vi "FL Gaussian COA Single Side.vi"(0 "weight":dbl, 5 "Implication":T1 items=["Minimum", "Product"]) -> (4 "xlh":dbl, 6 "area":dbl, 8 "coa_x":dbl, 10 "x_l":dbl=-2.5, 15 "x_r":dbl)   [LabVIEW 2017, in "NI_Fuzzy_Logic_API.lvlib"]
uses:
  <vilib>/addons/Fuzzy Logic/NI_Fuzzy_Logic_API.lvlib
  <vilib>/addons/Fuzzy Logic/TypeDefs/FL Consequent Implication.ctl
  <vilib>/gmath/NI_Gmath.lvlib
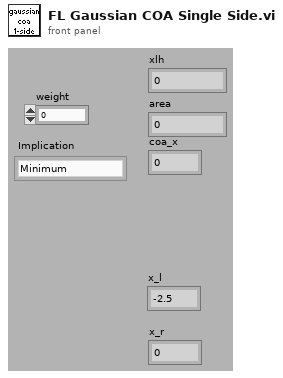
[diagram p1: front panel]
types:
  T1 = typedef "NI_Fuzzy_Logic_API.lvlib/FL Consequent Implication.ctl" = u16
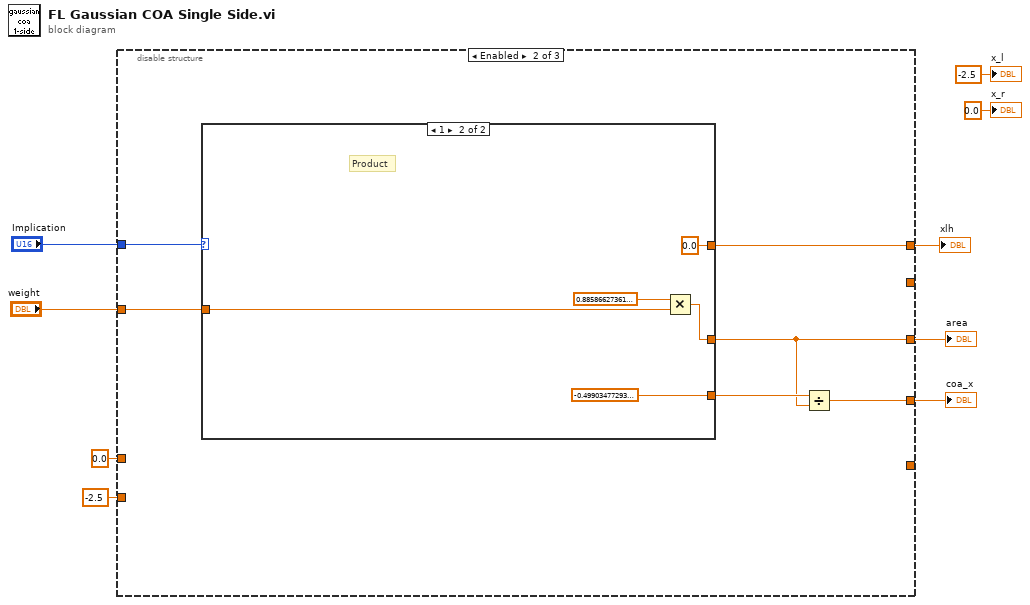
[diagram p0: block diagram]
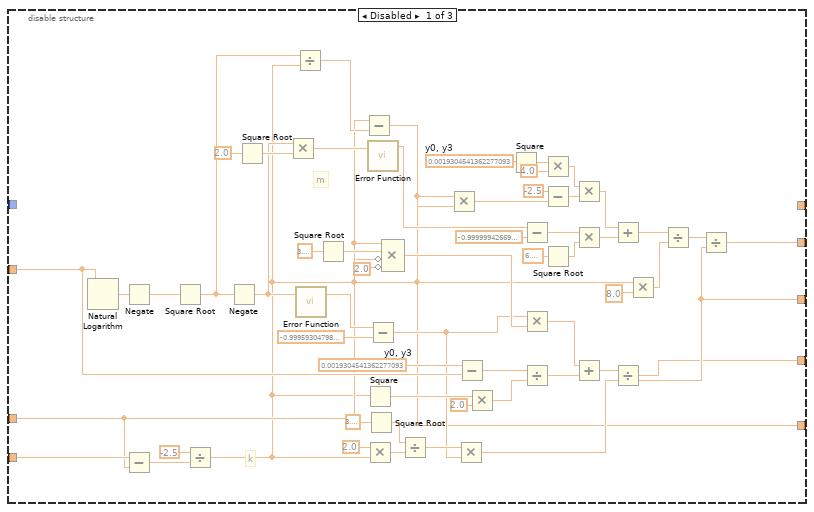
[diagram p2: hidden frame]
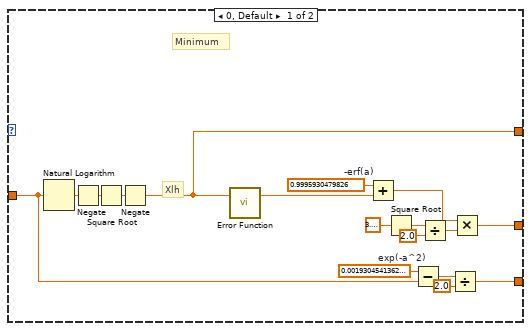
[diagram p3: hidden frame]
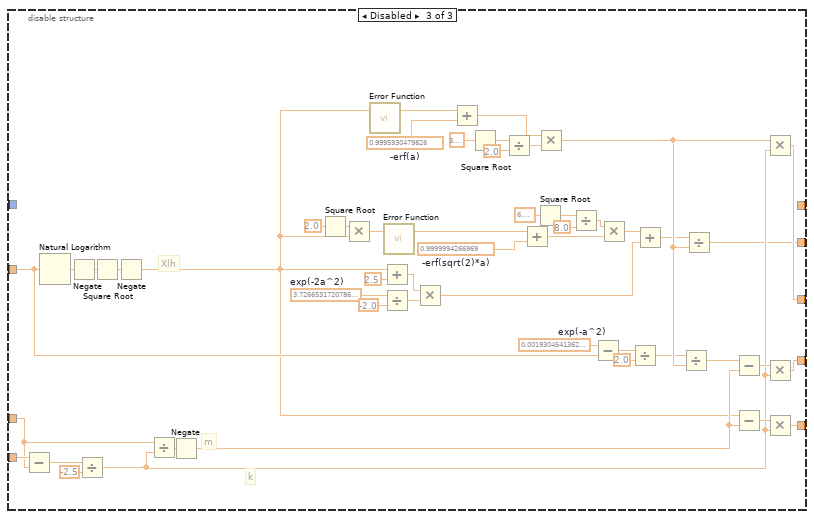
[diagram p4: hidden frame]
diagram:
  n1 = disable-structure shown="Enabled" {
    disable-tunnel: "weight" -> [w65 w70 w111]
    disable-tunnel: [w61 w69 w99] -> w8
    disable-tunnel: [w59 _ w96] -> _
    disable-tunnel: -2.5 ("x0") -> [w27 _ w133]
    disable-tunnel: 0.0 ("x1") -> [w15 _ w124]
    disable-tunnel: [w14 w68 w114] -> w7
    disable-tunnel: [w10 _ w121] -> _
    disable-tunnel: "Implication" -> [_ w67 _]
    disable-tunnel: [_ w66 _] -> w1
    frame Disabled {
      w13 = 0.0019304541362277093  # y0, y3
      w47 = 0.0019304541362277093  # y0, y3
      # "m"
      # "k"
      n2 = Natural Logarithm(1:w65) -> (0:w19:dbl)
      n3 = Negate(x=w19) -> (-x=w20:dbl)
      n4 = Subtract(x=w27, y=w15) -> (x-y=w18:dbl)
      n5 = Square Root(x=w20) -> (sqrt(x)=w64:dbl)
      n6 = Divide(x=-2.5, y=w18) -> (x/y=w12:dbl)
      n7 = Negate(x=w64) -> (-x=w38:dbl)
      n8 = Square Root(x=2.0) -> (sqrt(x)=w41:dbl)
      n9 = Multiply(x=w38, y=w41) -> (x*y=w40:dbl)
      n10 = Divide(x=w64, y=w12) -> (x/y=w21:dbl)
      n11 = call <vilib>:"Error Function.vi"("x"=w38) -> ("erf(x)"=w22:dbl)  [unwired: 2 out]
      n12 = Square Root(x=3.141592653589793) -> (sqrt(x)=w29:dbl)
      n13 = Subtract(x=w15, y=w21) -> (x-y=w10:dbl)
      n14 = Square(x=w12) -> (x^2=w32:dbl)
      n15 = Multiply(x=2.0, y=w12) -> (x*y=w25:dbl)
      n16 = Square Root(x=3.141592653589793) -> (sqrt(x)=w62:dbl)
      n17 = call <vilib>:"Error Function.vi"("x"=w40) -> ("erf(x)"=w42:dbl)  [unwired: 2 out]
      n18 = Subtract(x=w22, y=-0.999593047982555 ("erf(x)")) -> (x-y=w11:dbl)
      n19 = Compound Arithmetic op=MULTIPLY(w15, w29, invert w12, invert 2.0 ("value")) -> (w31:dbl)
      n20 = Divide(x=w62, y=w25) -> (x/y=w26:dbl)
      n21 = Multiply(x=w10, y=w12) -> (x*y=w51:dbl)
      n22 = Multiply(x=w26, y=w11) -> (x*y=w61:dbl)
      n23 = Subtract(x=w13, y=w65) -> (x-y=w34:dbl)
      n24 = Multiply(x=w32, y=2.0) -> (x*y=w35:dbl)
      n25 = Square(x=w47) -> (x^2=w48:dbl)
      n26 = Subtract(x=w42, y=-0.9999994266968563 ("erf(x)")) -> (x-y=w45:dbl)
      n27 = Multiply(x=w11, y=w31) -> (x*y=w37:dbl)
      n28 = Divide(x=w34, y=w35) -> (x/y=w36:dbl)
      n29 = Multiply(x=w48, y=4.0) -> (x*y=w50:dbl)
      n30 = Subtract(x=-2.5, y=w51) -> (x-y=w53:dbl)
      n31 = Square Root(x=6.283185307179586) -> (sqrt(x)=w46:dbl)
      n32 = Multiply(x=w50, y=w53) -> (x*y=w54:dbl)
      n33 = Multiply(x=w45, y=w46) -> (x*y=w55:dbl)
      n34 = Add(x=w37, y=w36) -> (x+y=w58:dbl)
      n35 = Add(x=w54, y=w55) -> (x+y=w57:dbl)
      n36 = Divide(x=w58, y=w61) -> (x/y=w14:dbl)
      n37 = Multiply(x=w12, y=8.0) -> (x*y=w63:dbl)
      n38 = Divide(x=w57, y=w63) -> (x/y=w60:dbl)
      n39 = Divide(x=w60, y=w61) -> (x/y=w59:dbl)
    }
    frame Enabled {
      n40 = case shown="1" w67 {
        tunnel: [w88 w90] -> w69
        tunnel: w70 -> [w75 w92]
        tunnel: [w73 -0.49903477293189] -> w71
        tunnel: [w72 0.0] -> w66
        frame 0, Default {
          w74 = 0.0019304541362277093  # exp(-a^2)
          w78 = 0.9995930479826  # -erf(a)
          # "Minimum"
          # "Xlh"
          n41 = Natural Logarithm(1:w75) -> (0:w81:dbl)
          n42 = Negate(x=w81) -> (-x=w82:dbl)
          n43 = Square Root(x=w82) -> (sqrt(x)=w77:dbl)
          n44 = Negate(x=w77) -> (-x=w72:dbl)
          n45 = call <vilib>:"Error Function.vi"("x"=w72) -> ("erf(x)"=w83:dbl)  [unwired: 2 out]
          n46 = Add(x=w78, y=w83) -> (x+y=w80:dbl)
          n47 = Square Root(x=3.141592653589793) -> (sqrt(x)=w87:dbl)
          n48 = Subtract(x=w74, y=w75) -> (x-y=w86:dbl)
          n49 = Divide(x=w87, y=2.0 ("x")) -> (x/y=w85:dbl)
          n50 = Divide(x=w86, y=2.0) -> (x/y=w73:dbl)
          n51 = Multiply(x=w80, y=w85) -> (x*y=w88:dbl)
        }
        frame 1 {
          # "Product"
          n52 = Multiply(x=0.88586627361757, y=w92) -> (x*y=w90:dbl)
        }
      }
      n53 = Divide(x=w71, y=w69) -> (x/y=w68:dbl)
    }
    frame Disabled {
      w98 = 0.0019304541362277093  # exp(-a^2)
      w104 = 3.7266531720786714e-06  # exp(-2a^2)
      w113 = 0.9999994266969  # -erf(sqrt(2)*a)
      w119 = 0.9995930479826  # -erf(a)
      # "Xlh"
      # "m"
      # "k"
      n54 = Subtract(x=w133, y=w124) -> (x-y=w127:dbl)
      n55 = Natural Logarithm(1:w111) -> (0:w128:dbl)
      n56 = Negate(x=w128) -> (-x=w129:dbl)
      n57 = Divide(x=w127, y=-2.5) -> (x/y=w100:dbl)
      n58 = Square Root(x=w129) -> (sqrt(x)=w118:dbl)
      n59 = Negate(x=w118) -> (-x=w108:dbl)
      n60 = Divide(x=w124, y=w100) -> (x/y=w123:dbl)
      n61 = Negate(x=w123) -> (-x=w115:dbl)
      n62 = Square Root(x=2.0) -> (sqrt(x)=w137:dbl)
      n63 = Multiply(x=w137, y=w108) -> (x*y=w136:dbl)
      n64 = call <vilib>:"Error Function.vi"("x"=w108) -> ("erf(x)"=w130:dbl)  [unwired: 2 out]
      n65 = Add(x=w108, y=2.5) -> (x+y=w106:dbl)
      n66 = Divide(x=w104, y=-2.0) -> (x/y=w109:dbl)
      n67 = call <vilib>:"Error Function.vi"("x"=w136) -> ("erf(x)"=w138:dbl)  [unwired: 2 out]
      n68 = Multiply(x=w106, y=w109) -> (x*y=w105:dbl)
      n69 = Add(x=w130, y=w119) -> (x+y=w125:dbl)
      n70 = Square Root(x=3.141592653589793) -> (sqrt(x)=w141:dbl)
      n71 = Divide(x=w141, y=2.0 ("x")) -> (x/y=w132:dbl)
      n72 = Add(x=w138, y=w113) -> (x+y=w140:dbl)
      n73 = Square Root(x=6.283185307179586) -> (sqrt(x)=w103:dbl)
      n74 = Multiply(x=w125, y=w132) -> (x*y=w142:dbl)
      n75 = Divide(x=w103, y=8.0) -> (x/y=w102:dbl)
      n76 = Subtract(x=w98, y=w111) -> (x-y=w134:dbl)
      n77 = Multiply(x=w102, y=w140) -> (x*y=w101:dbl)
      n78 = Divide(x=w134, y=2.0) -> (x/y=w95:dbl)
      n79 = Add(x=w101, y=w105) -> (x+y=w97:dbl)
      n80 = Divide(x=w95, y=w142) -> (x/y=w94:dbl)
      n81 = Divide(x=w97, y=w142) -> (x/y=w96:dbl)
      n82 = Subtract(x=w94, y=w115) -> (x-y=w116:dbl)
      n83 = Subtract(x=w108, y=w115) -> (x-y=w122:dbl)
      n84 = Multiply(x=w142, y=w100) -> (x*y=w99:dbl)
      n85 = Multiply(x=w116, y=w100) -> (x*y=w114:dbl)
      n86 = Multiply(x=w122, y=w100) -> (x*y=w121:dbl)
    }
  }
  "area" <- w8
  "coa_x" <- w7
  "xlh" <- w1
  "x_l" <- -2.5 ("x_l")
  "x_r" <- 0.0 ("x_r")
